vi "Save Device Settings to File.vi"(2 "Error In":errorcluster, 3 "Device Settings":T1={"Device Type"="", "Device Name"="", "DAQmx Name"="Dev1", "Terminal Wiring"=10106} {"Terminal Wiring" items=["Default"=-1, "RSE"=10083, "NRSE"=10078, "Differential"=10106, "Pseudodifferential"=12529]}) -> (0 "Error Out":errorcluster)   [LabVIEW 2019]
uses:
  Controls/Device Settings.ctl
  <vilib>/Utility/config.llb/Write Key (String).vi
  <vilib>/Utility/config.llb/NI_LVConfig.lvlib
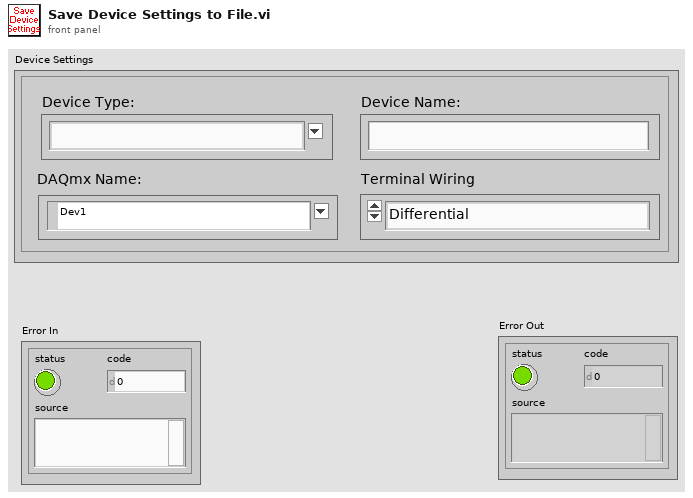
[diagram p1: front panel]
types:
  T1 = typedef "Device Settings.ctl" = cluster{"Device Type":string, "Device Name":string, "DAQmx Name":tag, "Terminal Wiring":i32}
  T2 = typedef "NI_LVConfig.lvlib/Config Data RefNum.ctl" = refnum<k1>
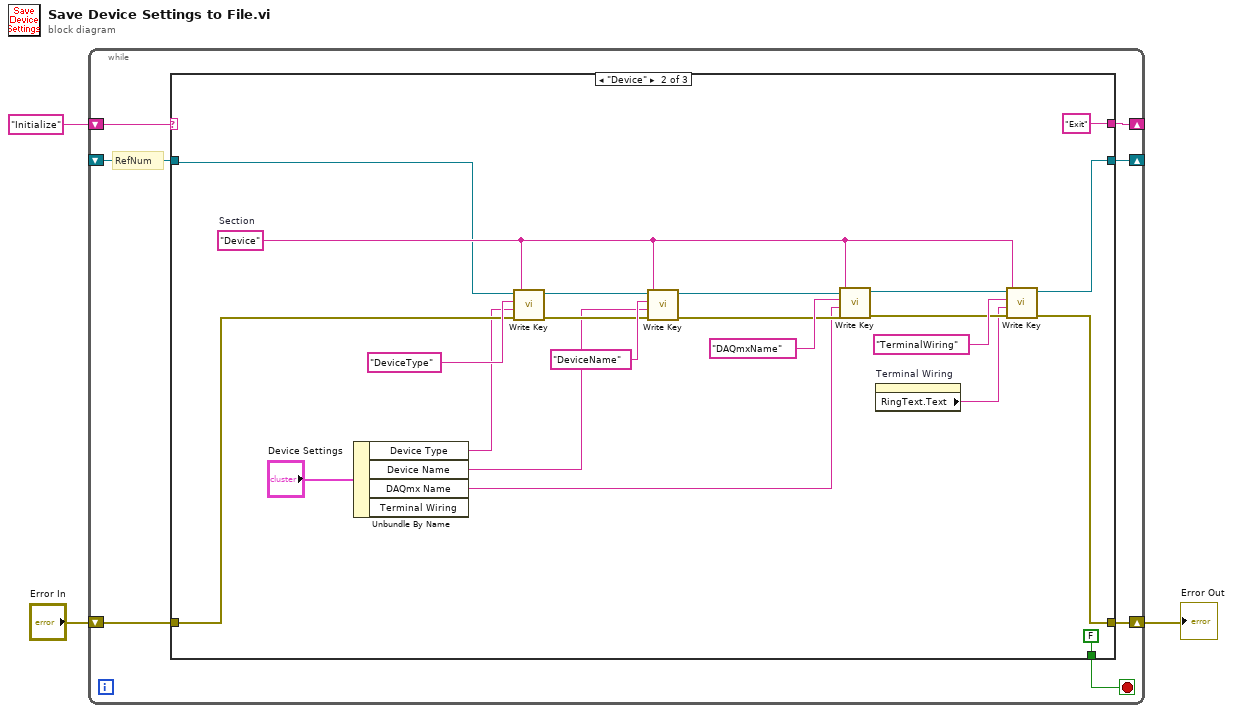
[diagram p0: block diagram]
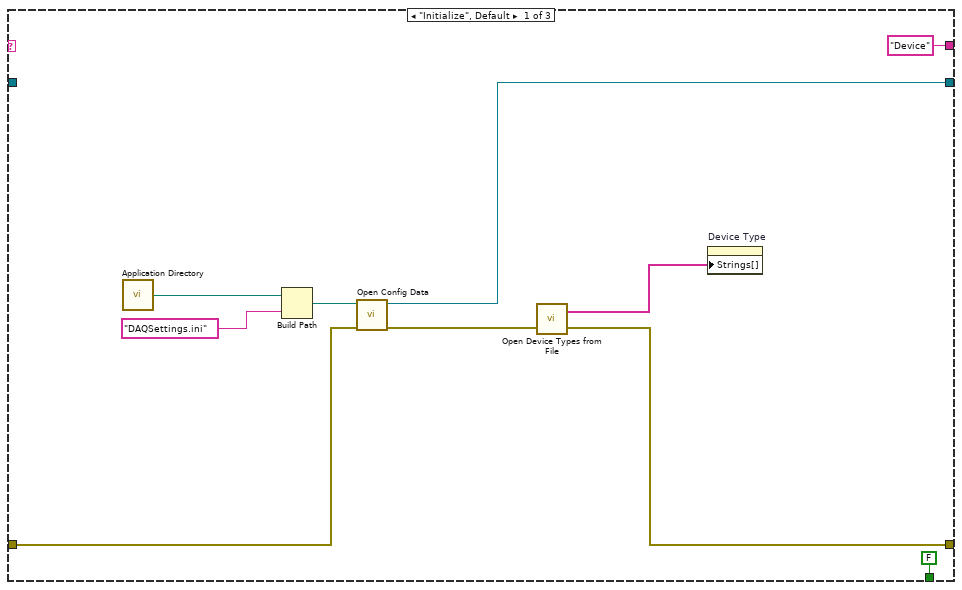
[diagram p2: hidden frame]
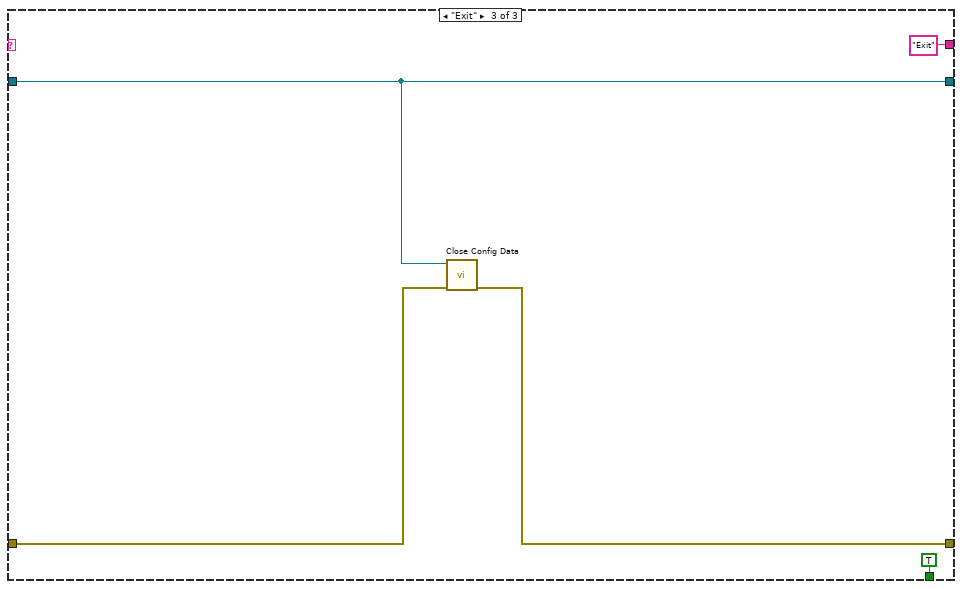
[diagram p3: hidden frame]
diagram:
  n1 = while {
    shift-right: [w5] -> _
    shift-left: "Initialize" ("key") -> [w10]
    shift-right: [w6] -> _
    shift-left: _ -> [w9]
    shift-right: [w7] -> w1
    shift-left: "Error In" -> [w8]
    stop <- w4 stop-if-true
    # "RefNum"
    n2 = case shown="\"Device\"" w10 {
      tunnel: w9 -> [_ w28 w45]
      tunnel: w8 -> [w20 w31 w47]
      tunnel: [w11 w38 w46] -> w7
      tunnel: [w19 w37 w45] -> w6
      tunnel: ["Device" ("key") "Exit" ("key") "Exit" ("key")] -> w5
      tunnel: [FALSE FALSE TRUE] -> w4
      frame "Initialize", Default {
        n3 = call <vilib>:"Application Directory.vi"() -> ("Application Directory"=w16:path)
        n4 = Build Path(base path=w16, name or relative path="DAQSettings.ini") -> (appended path=w14:path)
        n5 = call <vilib>:"Open Config Data.vi"("error in (no error)"=w20, "configuration file path"=w14) -> ("error out"=w12:errorcluster, "refnum"=w19:T2)  [unwired: 7 in, 1 out]
        n6 = call "Open Device Types from File.vi"("Error In"=w12) -> ("Error Out"=w11:errorcluster, "Device Types"=w13:string[])  [unwired: 1 in]
        n7 = property on="Device Type" class="CmbBox"("Strings[]"=w13) -> ()  [unwired: 2 in, 2 out]
      }
      frame "Device" {
        w32 = "Device"  # Section
        n8 = Unbundle By Name("Device Settings") -> ("Device Type"=w21:string, "Device Name"=w24:string, "DAQmx Name"=w23:tag)  [unwired: 1 out]
        n9 = call-poly <vilib>:"Write Key.vi"("section"=w32, "error in (no error)"=w31, "value"=w21, "key"="DeviceType", "refnum"=w28) -> ("error out"=w30:errorcluster, "refnum out"=w27:T2)  [unwired: 4 in, 1 out]
        n10 = call-poly <vilib>:"Write Key.vi"("section"=w32, "error in (no error)"=w30, "value"=w24, "key"="DeviceName", "refnum"=w27) -> ("error out"=w29:errorcluster, "refnum out"=w26:T2)  [unwired: 4 in, 1 out]
        n11 = call-poly <vilib>:"Write Key.vi"("section"=w32, "error in (no error)"=w29, "value"=w23, "key"="DAQmxName", "refnum"=w26) -> ("error out"=w41:errorcluster, "refnum out"=w40:T2)  [unwired: 4 in, 1 out]
        n12 = property on="Terminal Wiring" class="Ring (strict)"() -> ("RingText.Text"=w22:string)  [unwired: 2 in, 2 out]
        n13 = call-poly <vilib>:"Write Key.vi"("section"=w32, "error in (no error)"=w41, "value"=w22, "key"="TerminalWiring", "refnum"=w40) -> ("error out"=w38:errorcluster, "refnum out"=w37:T2)  [unwired: 4 in, 1 out]
      }
      frame "Exit" {
        n14 = call <vilib>:"Close Config Data.vi"("error in (no error)"=w47, "refnum"=w45) -> ("error out"=w46:errorcluster)  [unwired: 8 in, 1 out]
      }
    }
  }
  "Error Out" <- w1
